vi "MPUReadData.vi"(8 "ErrorIn":errorcluster caption="错误输入", 11 "FPGA VI引用输入":refnum<k20>) -> (0 "ErrorOut":errorcluster caption="error IO", 1 "GYR":cluster{"GYR_X":i16, "GYR_Y":i16, "GYR_Z":i16}, 2 "ACC":cluster{"ACC_X":i16, "ACC_Y":i16, "ACC_Z":i16}, 3 "FPGA VI引用输出":refnum<k20>, 5 "TEMP":i16)   [LabVIEW 2015]
uses:
  <vilib>/Utility/error.llb/Error Cluster From Error Code.vi
  <vilib>/rvi/errors/niLvFpgaAdjustHostInterfaceError.vi
  <vilib>/rvi/interface/nirviReadWriteControl/nirviReadWriteControl.xnode
  NiFpgaLv.dll
  <vilib>/rvi/interface/Simulation/niFpgaSimulationCallBeginRW.vi
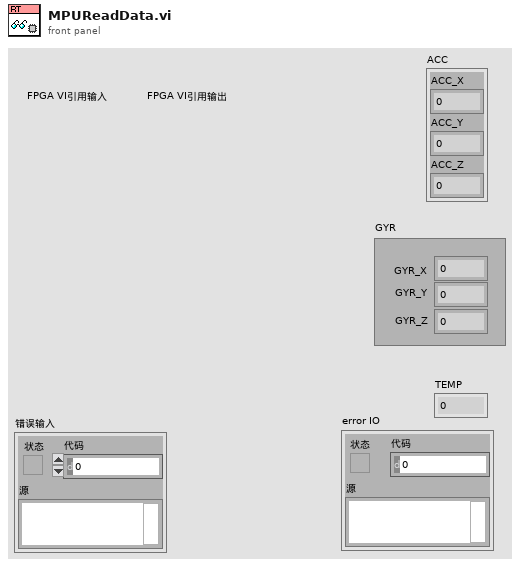
[diagram p1: front panel]
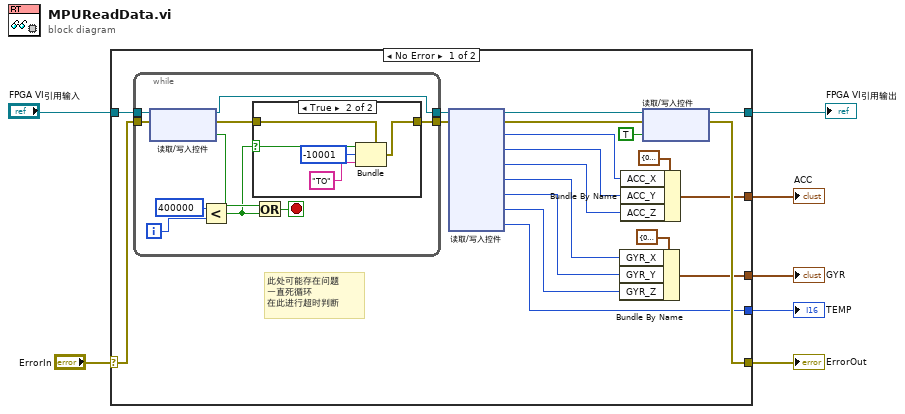
[diagram p0: block diagram]
diagram:
  n1 = case shown="No Error" "ErrorIn" {
    selector: "ErrorIn" -> [w26 w44]
    tunnel: "FPGA VI引用输入" -> [w27 w45]
    tunnel: [w20 w45] -> w1
    tunnel: [w19 w44] -> w6
    tunnel: [w10 _] -> w5
    tunnel: [w9 _] -> w4
    tunnel: [w8 _] -> w3
    frame No Error {
      # "此处可能存在问题\n一直死循环\n在此进行超时判断"
      n2 = while {
        tunnel: w27 -> [w37]
        tunnel: w26 -> [w36]
        tunnel: [w35] -> w25
        tunnel: [w31] -> w24
        i -> [w34]
        stop <- w29 stop-if-true
        n3 = xnode "读取/写入控件"("FPGA VI Reference In"=w37, "error in"=w36) -> ("FPGA VI Reference Out"=w35:refnum<k20>, "error out"=w32:errorcluster, "DataAva"=w30:bool)
        n4 = Less?(x=400000, y=w34) -> (x < y?=w28:bool)
        n5 = case shown="True" w28 {
          selector: w28 -> [_ w39]
          tunnel: w32 -> [w38 w43]
          tunnel: [w38 w42] -> w31
          frame False {
          }
          frame True {
            n6 = Bundle(cluster=w43, "status"=w39, "code"=-10001, "source"="TO") -> (w42:errorcluster)
          }
        }
        n7 = Or(x=w30, y=w28) -> (x .or. y?=w29:bool)
      }
      n8 = xnode "读取/写入控件"("FPGA VI Reference In"=w25, "error in"=w24) -> ("FPGA VI Reference Out"=w23:refnum<k20>, "error out"=w22:errorcluster, "ACC_X"=w17:i16, "ACC_Y"=w16:i16, "ACC_Z"=w15:i16, "GYR_X"=w13:i16, "GYR_Y"=w12:i16, "GYR_Z"=w11:i16, "TEMP"=w9:i16)
      n9 = Bundle By Name(cluster=cluster{"GYR_X":i16, "GYR_Y":i16, "GYR_Z":i16} {"GYR_X"=0, "GYR_Y"=0, "GYR_Z"=0} ("GYR"), "GYR_X"=w13, "GYR_Y"=w12, "GYR_Z"=w11) -> (w10:cluster{"GYR_X":i16, "GYR_Y":i16, "GYR_Z":i16})
      n10 = Bundle By Name(cluster=cluster{"ACC_X":i16, "ACC_Y":i16, "ACC_Z":i16} {"ACC_X"=0, "ACC_Y"=0, "ACC_Z"=0} ("ACC"), "ACC_X"=w17, "ACC_Y"=w16, "ACC_Z"=w15) -> (w8:cluster{"ACC_X":i16, "ACC_Y":i16, "ACC_Z":i16})
      n11 = xnode "读取/写入控件"("FPGA VI Reference In"=w23, "error in"=w22, "DataAva"=TRUE) -> ("FPGA VI Reference Out"=w20:refnum<k20>, "error out"=w19:errorcluster)
    }
    frame Error {
    }
  }
  "ErrorOut" <- w6
  "TEMP" <- w4
  "GYR" <- w5
  "ACC" <- w3
  "FPGA VI引用输出" <- w1
